vi "Configure Voltage Range.vi"(0 "VISA resource name":refnum<visa-resource-name>, 2 "Enable Auto Range (F: Disable)":bool, 5 "Range Configuration (True)":bool[](array[boolean])=[TRUE, TRUE, TRUE, TRUE, TRUE, TRUE, TRUE, TRUE, TRUE, TRUE, TRUE, TRUE], 7 "Enable Peak Over Jump (F: Disable)":bool, 9 "Jump Range (600 <300> V)":dbl(ring)=300.0 items=["15 <7.5>"=7.5, "30 <15>"=15.0, "60 <30>"=30.0, "150 <75>"=75.0, "300 <150>"=150.0, "600 <300>"=300.0], 11 "error in (no error)":errorcluster, 12 "Manual Range (600 <300> V)":dbl(ring)=300.0 items=["15 <7.5>"=7.5, "30 <15>"=15.0, "60 <30>"=30.0, "150 <75>"=75.0, "300 <150>"=150.0, "600 <300>"=300.0]) -> (4 "VISA resource name out":refnum<visa-resource-name>, 15 "error out":errorcluster)   [LabVIEW 2018, in "Yokogawa WT300 Series.lvlib"]
doc: "Configures the voltage range features."
uses:
  Yokogawa WT300 Series.lvlib
panel:
  # "15 <7.5> V"
  # "30 <15> V"
  # "60 <30> V"
  # "150 <75> V"
  # "300 <150> V"
  # "600 <300> V"
  # "V"
  # "V"
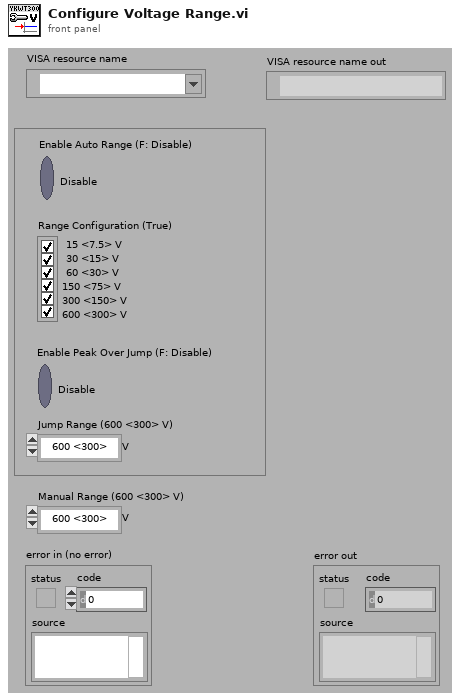
[diagram p1: front panel]
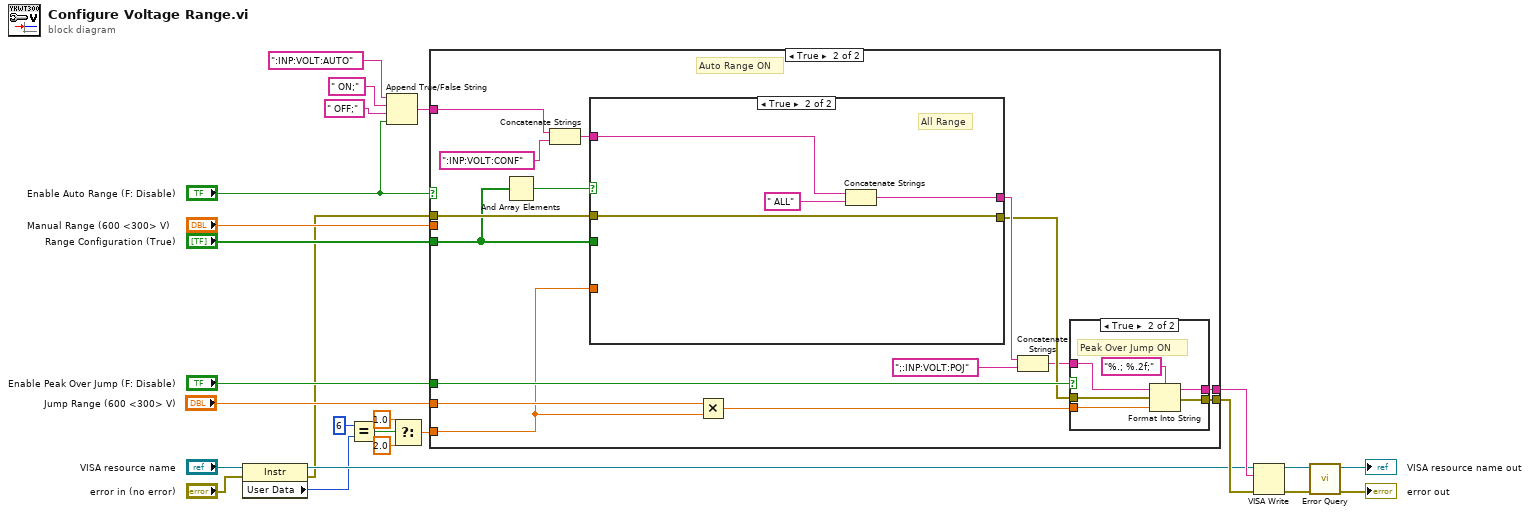
[diagram p0: block diagram]
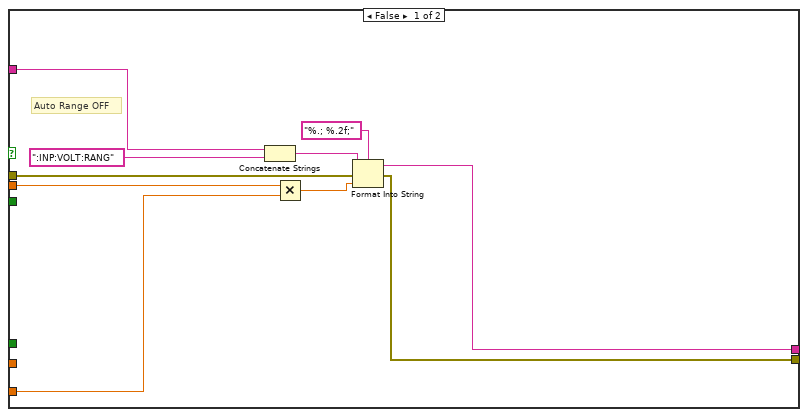
[diagram p2: hidden frame]
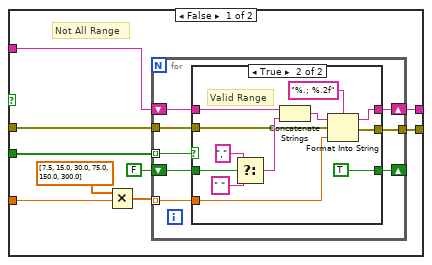
[diagram p3: hidden frame]
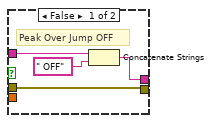
[diagram p5: hidden frame]
diagram:
  n1 = property class="Instr"(reference="VISA resource name", error in="error in (no error)") -> (reference out=w4:refnum<visa-resource-name>, error out=w3:errorcluster, "User Data"=w2:u32)
  n2 = Equal?(x=i64 6 ("y"), y=w2) -> (x = y?=w15:bool)
  n3 = Append True/False String ("True/False 文字列を追加")(1:"Enable Auto Range (F: Disable)", 2:" OFF;", 3:" ON;", 4:":INP:VOLT:AUTO") -> (0:w11:string)
  n4 = Select(t=1.0 ("y"), s=w15, f=2.0 ("y")) -> (s? t:f=w13:dbl)
  n5 = case shown="True" "Enable Auto Range (F: Disable)" {
    tunnel: "Manual Range (600 <300> V)" -> [w32 _]
    tunnel: w13 -> [w31 w38]
    tunnel: "Range Configuration (True)" -> [_ w40]
    tunnel: w11 -> [w30 w43]
    tunnel: "Enable Peak Over Jump (F: Disable)" -> [_ w50]
    tunnel: "Jump Range (600 <300> V)" -> [_ w47]
    tunnel: [w29 w49] -> w8
    tunnel: w3 -> [w28 w46]
    tunnel: [w27 w45] -> w7
    frame False {
      # "Auto Range OFF"
      n6 = Concatenate Strings(w30, ":INP:VOLT:RANG") -> (w35:string)
      n7 = Multiply(x=w32, y=w31) -> (x*y=w33:dbl)
      n8 = Format Into String(format string="%.; %.2f;" ("Œ`Ž®•¶Žš—ñ"), initial string=w35, error in=w28, w33) -> (resulting string=w29:string, error out=w27:errorcluster)
    }
    frame True {
      # "Auto Range ON"
      n9 = And Array Elements(Boolean array=w40) -> (logical AND=w39:bool)
      n10 = Concatenate Strings(w43, ":INP:VOLT:CONF") -> (w41:string)
      n11 = case shown="True" w39 {
        tunnel: w40 -> [w60 _]
        tunnel: w38 -> [w53 _]
        tunnel: [w59 w84] -> w51
        tunnel: w46 -> [w58 w87]
        tunnel: [w57 w87] -> w44
        tunnel: w41 -> [w55 w85]
        frame False {
          # "Not All Range"
          n12 = Multiply(x=dbl[] [7.5, 15.0, 30.0, 75.0, 150.0, 300.0], y=w53) -> (x*y=w52:dbl[])
          n13 = for {
            tunnel: w60 -> [w66] mode=indexing
            shift-right: [w67] -> w59
            shift-left: w55 -> [w68]
            tunnel: w52 -> [w65] mode=indexing
            tunnel: w58 -> [w64]
            tunnel: [w63] -> w57
            shift-right: [w61] -> _
            shift-left: FALSE -> [w62]
            n14 = case shown="True" w66 {
              tunnel: w68 -> [w71 w81]
              tunnel: [w71 w77] -> w67
              tunnel: w65 -> [_ w76]
              tunnel: w64 -> [w70 w75]
              tunnel: [w70 w74] -> w63
              tunnel: w62 -> [w69 w73]
              tunnel: [w69 TRUE] -> w61
              frame False {
                # "Invalid Range"
              }
              frame True {
                # "Valid Range"
                n15 = Select(t=",", s=w73, f=" ") -> (s? t:f=w80:string)
                n16 = Concatenate Strings(w81, w80) -> (w79:string)
                n17 = Format Into String(format string="%.; %.2f" ("Œ`Ž®•¶Žš—ñ"), initial string=w79, error in=w75, w76) -> (resulting string=w77:string, error out=w74:errorcluster)
              }
            }
          }
        }
        frame True {
          # "All Range"
          n18 = Concatenate Strings(w85, " ALL") -> (w84:string)
        }
      }
      n19 = Multiply(x=w47, y=w38) -> (x*y=w48:dbl)
      n20 = Concatenate Strings(w51, ";:INP:VOLT:POJ") -> (w37:string)
      n21 = case shown="True" w50 {
        tunnel: w37 -> [w90 w96]
        tunnel: w48 -> [_ w95]
        tunnel: [w89 w94] -> w49
        tunnel: [w88 w93] -> w45
        tunnel: w44 -> [w88 w92]
        frame False {
          # "Peak Over Jump OFF"
          n22 = Concatenate Strings(w90, " OFF" ("•¶Žš—ñ")) -> (w89:string)
        }
        frame True {
          # "Peak Over Jump ON"
          n23 = Format Into String(format string="%.; %.2f;" ("Œ`Ž®•¶Žš—ñ"), initial string=w96, error in=w92, w95) -> (resulting string=w94:string, error out=w93:errorcluster)
        }
      }
    }
  }
  n24 = VISA Write ("VISA書き込み")(VISA resource name=w4, write buffer=w8, error in (no error)=w7) -> (VISA resource name out=w25:refnum<visa-resource-name>, error out=w24:errorcluster)  [unwired: 1 out]
  n25 = call "Error Query.vi"("error in (no error)"=w24, "VISA resource name"=w25) -> ("error out"=→"error out":errorcluster, "VISA resource name out"=→"VISA resource name out":refnum<visa-resource-name>)  [unwired: 6 in, 2 out]
